vi "Scope signal frame trim.vi"(0 "Waveform Data":waveform(dbl), 5 "Frame delete":i32=5, 7 "offset":dbl format="%#_13g", 9 "start/duration format":u16(ring) items=["Samples", "Relative Time"], 11 "error in (no error)":errorcluster) -> (4 "waveform out":waveform(dbl), 15 "error out":errorcluster)   [LabVIEW 2018]
uses:
  <vilib>/Waveform/WDTOps.llb/WDT Get Waveform Subset DBL.vi
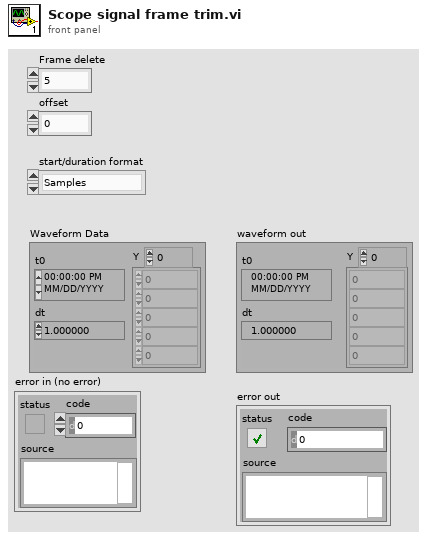
[diagram p1: front panel]
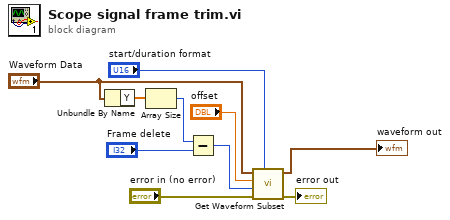
[diagram p0: block diagram]
diagram:
  n1 = Unbundle By Name("Waveform Data") -> ("Y"=w6:dbl[])
  n2 = Array Size(array=w6) -> (size(s)=w8:i32)
  n3 = Subtract(x=w8, y="Frame delete") -> (x-y=w7:i32)
  n4 = call-poly <vilib>:"Get Waveform Subset.vi"("start/duration format"="start/duration format", "error in (no error)"="error in (no error)", "duration"=w7, "start samples/time"="offset", "waveform in"="Waveform Data") -> ("error out"=→"error out":errorcluster, "waveform out"=→"waveform out":waveform(dbl))  [unwired: 1 in, 2 out]
